vi "TSLIN_LIN_Tab.vi"(7 "Fold Data":bool, 8 "error in (no error)":errorcluster, 9 "Data in":T1 {"REC_Channel" items=["CHN1", "CHN2", "CHN3", "CHN4", "CHN5", "CHN6", "CHN7", "CHN8", "CHN9", "CHN10", "CHN11", "CHN12", "CHN13", "CHN14", "CHN15", "CHN16", "CHN17", "CHN18", "CHN19", "CHN20", "CHN21", "CHN22", "CHN23", "CHN24", "CHN25", "CHN26", "CHN27", "CHN28", "CHN29", "CHN30", "CHN31", "CHN32"]; "LIN_Data"."REC_Channel" items=["CHN1", "CHN2", "CHN3", "CHN4", "CHN5", "CHN6", "CHN7", "CHN8", "CHN9", "CHN10", "CHN11", "CHN12", "CHN13", "CHN14", "CHN15", "CHN16", "CHN17", "CHN18", "CHN19", "CHN20", "CHN21", "CHN22", "CHN23", "CHN24", "CHN25", "CHN26", "CHN27", "CHN28", "CHN29", "CHN30", "CHN31", "CHN32"]; "LIN_Data"."LIN Scheduling Table Array"."LIN_Transmit"."Channel" items=["CHN1", "CHN2", "CHN3", "CHN4", "CHN5", "CHN6", "CHN7", "CHN8", "CHN9", "CHN10", "CHN11", "CHN12", "CHN13", "CHN14", "CHN15", "CHN16", "CHN17", "CHN18", "CHN19", "CHN20", "CHN21", "CHN22", "CHN23", "CHN24", "CHN25", "CHN26", "CHN27", "CHN28", "CHN29", "CHN30", "CHN31", "CHN32"]; "LIN_Data"."LIN Scheduling Table Array"."LIN_Transmit"."ID" format="%.0x"; "LIN_Data"."LIN Scheduling Table Array"."LIN_Transmit"."DLC" format="%.0x"; "LIN_Data"."LIN Scheduling Table Array"."LIN_Transmit"."Set_node_funtiontype" items=["MasterNode", "SlaveNode", "MonitorNote"]; "LIN_Data"."LDF"."LDF loading channel" items=["CHN1", "CHN2", "CHN3", "CHN4", "CHN5", "CHN6", "CHN7", "CHN8", "CHN9", "CHN10", "CHN11", "CHN12", "CHN13", "CHN14", "CHN15", "CHN16", "CHN17", "CHN18", "CHN19", "CHN20", "CHN21", "CHN22", "CHN23", "CHN24", "CHN25", "CHN26", "CHN27", "CHN28", "CHN29", "CHN30", "CHN31", "CHN32"]; "LIN_Data"."LIN_Set_Array"."Set_node_funtiontype" items=["MasterNode", "SlaveNode", "MonitorNote"]; "LIN_Data"."LIN_Set_Array"."Set"."Hardware Type" items=["BUS_UNKNOWN_TYPE", "TS_TCP_DEVICE", "XL_USB_DEVICE", "TS_USB_DEVICE", "PEAK_USB_DEVICE", "KVASER_USB_DEVICE", "ZLG_USB_DEVICE", "ICS_USB_DEVICE", "TS_TC1005_DEVICE", "CANABLE_USB_DEVICE", "TS_WIRELESS_OBD", "TS_USB_DEVICE_EX", "IXXAT_USB_DEVICE", "TS_ETH_IF_DEVICE", "TS_USB_IF_DEVICE", "BUS_DEV_TYPE_COUNT"]; "LIN_Data"."LIN_Set_Array"."Set"."AHwChannel" items=["CHN1", "CHN2", "CHN3", "CHN4", "CHN5", "CHN6", "CHN7", "CHN8", "CHN9", "CHN10", "CHN11", "CHN12", "CHN13", "CHN14", "CHN15", "CHN16", "CHN17", "CHN18", "CHN19", "CHN20", "CHN21", "CHN22", "CHN23", "CHN24", "CHN25", "CHN26", "CHN27", "CHN28", "CHN29", "CHN30", "CHN31", "CHN32"]; "LIN_Data"."LIN_Set_Array"."Set"."AAppChannel" items=["CHN1", "CHN2", "CHN3", "CHN4", "CHN5", "CHN6", "CHN7", "CHN8", "CHN9", "CHN10", "CHN11", "CHN12", "CHN13", "CHN14", "CHN15", "CHN16", "CHN17", "CHN18", "CHN19", "CHN20", "CHN21", "CHN22", "CHN23", "CHN24", "CHN25", "CHN26", "CHN27", "CHN28", "CHN29", "CHN30", "CHN31", "CHN32"]; "LIN_Data"."LIN_Set_Array"."Set"."AProtocol" items=["Lin_Protocol_13", "Lin_Protocol_20", "Lin_Protocol_21", "Lin_Protocol_J2602"]; "LIN_Data"."Funtiontype" items=["MasterNode", "SlaveNode", "MonitorNote"]; "LIN_Data"."LIN_SendHead"."ALINDLC" format="%.0x"; "LIN_Data"."LIN_SendHead"."ALINId" format="%.0x"; "LIN_Data"."LIN_SendHead"."ALINIdxchn" items=["CHN1", "CHN2", "CHN3", "CHN4", "CHN5", "CHN6", "CHN7", "CHN8", "CHN9", "CHN10", "CHN11", "CHN12", "CHN13", "CHN14", "CHN15", "CHN16", "CHN17", "CHN18", "CHN19", "CHN20", "CHN21", "CHN22", "CHN23", "CHN24", "CHN25", "CHN26", "CHN27", "CHN28", "CHN29", "CHN30", "CHN31", "CHN32"]; "LIN_Data"."LIN_Set"."Hardware Type" items=["BUS_UNKNOWN_TYPE", "TS_TCP_DEVICE", "XL_USB_DEVICE", "TS_USB_DEVICE", "PEAK_USB_DEVICE", "KVASER_USB_DEVICE", "ZLG_USB_DEVICE", "ICS_USB_DEVICE", "TS_TC1005_DEVICE", "CANABLE_USB_DEVICE", "TS_WIRELESS_OBD", "TS_USB_DEVICE_EX", "IXXAT_USB_DEVICE", "TS_ETH_IF_DEVICE", "TS_USB_IF_DEVICE", "BUS_DEV_TYPE_COUNT"]; "LIN_Data"."LIN_Set"."AHwChannel" items=["CHN1", "CHN2", "CHN3", "CHN4", "CHN5", "CHN6", "CHN7", "CHN8", "CHN9", "CHN10", "CHN11", "CHN12", "CHN13", "CHN14", "CHN15", "CHN16", "CHN17", "CHN18", "CHN19", "CHN20", "CHN21", "CHN22", "CHN23", "CHN24", "CHN25", "CHN26", "CHN27", "CHN28", "CHN29", "CHN30", "CHN31", "CHN32"]; "LIN_Data"."LIN_Set"."AAppChannel" items=["CHN1", "CHN2", "CHN3", "CHN4", "CHN5", "CHN6", "CHN7", "CHN8", "CHN9", "CHN10", "CHN11", "CHN12", "CHN13", "CHN14", "CHN15", "CHN16", "CHN17", "CHN18", "CHN19", "CHN20", "CHN21", "CHN22", "CHN23", "CHN24", "CHN25", "CHN26", "CHN27", "CHN28", "CHN29", "CHN30", "CHN31", "CHN32"]; "LIN_Data"."LIN_Set"."AProtocol" items=["Lin_Protocol_13", "Lin_Protocol_20", "Lin_Protocol_21", "Lin_Protocol_J2602"]; "LIN_Data"."Channels used" items=["1 Channel"=1, "2 Channels"=2, "3 Channels"=3, "4 Channels"=4, "5 Channels"=5]}, 10 "ALINBuffer":T11[](array[typedef]) {"Properties" format="%x"}, 11 "MulticolumnListbox in":refnum<vi>) -> (3 "Data out":T1 {"REC_Channel" items=["CHN1", "CHN2", "CHN3", "CHN4", "CHN5", "CHN6", "CHN7", "CHN8", "CHN9", "CHN10", "CHN11", "CHN12", "CHN13", "CHN14", "CHN15", "CHN16", "CHN17", "CHN18", "CHN19", "CHN20", "CHN21", "CHN22", "CHN23", "CHN24", "CHN25", "CHN26", "CHN27", "CHN28", "CHN29", "CHN30", "CHN31", "CHN32"]; "LIN_Data"."REC_Channel" items=["CHN1", "CHN2", "CHN3", "CHN4", "CHN5", "CHN6", "CHN7", "CHN8", "CHN9", "CHN10", "CHN11", "CHN12", "CHN13", "CHN14", "CHN15", "CHN16", "CHN17", "CHN18", "CHN19", "CHN20", "CHN21", "CHN22", "CHN23", "CHN24", "CHN25", "CHN26", "CHN27", "CHN28", "CHN29", "CHN30", "CHN31", "CHN32"]; "LIN_Data"."LIN Scheduling Table Array"."LIN_Transmit"."Channel" items=["CHN1", "CHN2", "CHN3", "CHN4", "CHN5", "CHN6", "CHN7", "CHN8", "CHN9", "CHN10", "CHN11", "CHN12", "CHN13", "CHN14", "CHN15", "CHN16", "CHN17", "CHN18", "CHN19", "CHN20", "CHN21", "CHN22", "CHN23", "CHN24", "CHN25", "CHN26", "CHN27", "CHN28", "CHN29", "CHN30", "CHN31", "CHN32"]; "LIN_Data"."LIN Scheduling Table Array"."LIN_Transmit"."ID" format="%.0x"; "LIN_Data"."LIN Scheduling Table Array"."LIN_Transmit"."DLC" format="%.0x"; "LIN_Data"."LIN Scheduling Table Array"."LIN_Transmit"."Set_node_funtiontype" items=["MasterNode", "SlaveNode", "MonitorNote"]; "LIN_Data"."LDF"."LDF loading channel" items=["CHN1", "CHN2", "CHN3", "CHN4", "CHN5", "CHN6", "CHN7", "CHN8", "CHN9", "CHN10", "CHN11", "CHN12", "CHN13", "CHN14", "CHN15", "CHN16", "CHN17", "CHN18", "CHN19", "CHN20", "CHN21", "CHN22", "CHN23", "CHN24", "CHN25", "CHN26", "CHN27", "CHN28", "CHN29", "CHN30", "CHN31", "CHN32"]; "LIN_Data"."LIN_Set_Array"."Set_node_funtiontype" items=["MasterNode", "SlaveNode", "MonitorNote"]; "LIN_Data"."LIN_Set_Array"."Set"."Hardware Type" items=["BUS_UNKNOWN_TYPE", "TS_TCP_DEVICE", "XL_USB_DEVICE", "TS_USB_DEVICE", "PEAK_USB_DEVICE", "KVASER_USB_DEVICE", "ZLG_USB_DEVICE", "ICS_USB_DEVICE", "TS_TC1005_DEVICE", "CANABLE_USB_DEVICE", "TS_WIRELESS_OBD", "TS_USB_DEVICE_EX", "IXXAT_USB_DEVICE", "TS_ETH_IF_DEVICE", "TS_USB_IF_DEVICE", "BUS_DEV_TYPE_COUNT"]; "LIN_Data"."LIN_Set_Array"."Set"."AHwChannel" items=["CHN1", "CHN2", "CHN3", "CHN4", "CHN5", "CHN6", "CHN7", "CHN8", "CHN9", "CHN10", "CHN11", "CHN12", "CHN13", "CHN14", "CHN15", "CHN16", "CHN17", "CHN18", "CHN19", "CHN20", "CHN21", "CHN22", "CHN23", "CHN24", "CHN25", "CHN26", "CHN27", "CHN28", "CHN29", "CHN30", "CHN31", "CHN32"]; "LIN_Data"."LIN_Set_Array"."Set"."AAppChannel" items=["CHN1", "CHN2", "CHN3", "CHN4", "CHN5", "CHN6", "CHN7", "CHN8", "CHN9", "CHN10", "CHN11", "CHN12", "CHN13", "CHN14", "CHN15", "CHN16", "CHN17", "CHN18", "CHN19", "CHN20", "CHN21", "CHN22", "CHN23", "CHN24", "CHN25", "CHN26", "CHN27", "CHN28", "CHN29", "CHN30", "CHN31", "CHN32"]; "LIN_Data"."LIN_Set_Array"."Set"."AProtocol" items=["Lin_Protocol_13", "Lin_Protocol_20", "Lin_Protocol_21", "Lin_Protocol_J2602"]; "LIN_Data"."Funtiontype" items=["MasterNode", "SlaveNode", "MonitorNote"]; "LIN_Data"."LIN_SendHead"."ALINDLC" format="%.0x"; "LIN_Data"."LIN_SendHead"."ALINId" format="%.0x"; "LIN_Data"."LIN_SendHead"."ALINIdxchn" items=["CHN1", "CHN2", "CHN3", "CHN4", "CHN5", "CHN6", "CHN7", "CHN8", "CHN9", "CHN10", "CHN11", "CHN12", "CHN13", "CHN14", "CHN15", "CHN16", "CHN17", "CHN18", "CHN19", "CHN20", "CHN21", "CHN22", "CHN23", "CHN24", "CHN25", "CHN26", "CHN27", "CHN28", "CHN29", "CHN30", "CHN31", "CHN32"]; "LIN_Data"."LIN_Set"."Hardware Type" items=["BUS_UNKNOWN_TYPE", "TS_TCP_DEVICE", "XL_USB_DEVICE", "TS_USB_DEVICE", "PEAK_USB_DEVICE", "KVASER_USB_DEVICE", "ZLG_USB_DEVICE", "ICS_USB_DEVICE", "TS_TC1005_DEVICE", "CANABLE_USB_DEVICE", "TS_WIRELESS_OBD", "TS_USB_DEVICE_EX", "IXXAT_USB_DEVICE", "TS_ETH_IF_DEVICE", "TS_USB_IF_DEVICE", "BUS_DEV_TYPE_COUNT"]; "LIN_Data"."LIN_Set"."AHwChannel" items=["CHN1", "CHN2", "CHN3", "CHN4", "CHN5", "CHN6", "CHN7", "CHN8", "CHN9", "CHN10", "CHN11", "CHN12", "CHN13", "CHN14", "CHN15", "CHN16", "CHN17", "CHN18", "CHN19", "CHN20", "CHN21", "CHN22", "CHN23", "CHN24", "CHN25", "CHN26", "CHN27", "CHN28", "CHN29", "CHN30", "CHN31", "CHN32"]; "LIN_Data"."LIN_Set"."AAppChannel" items=["CHN1", "CHN2", "CHN3", "CHN4", "CHN5", "CHN6", "CHN7", "CHN8", "CHN9", "CHN10", "CHN11", "CHN12", "CHN13", "CHN14", "CHN15", "CHN16", "CHN17", "CHN18", "CHN19", "CHN20", "CHN21", "CHN22", "CHN23", "CHN24", "CHN25", "CHN26", "CHN27", "CHN28", "CHN29", "CHN30", "CHN31", "CHN32"]; "LIN_Data"."LIN_Set"."AProtocol" items=["Lin_Protocol_13", "Lin_Protocol_20", "Lin_Protocol_21", "Lin_Protocol_J2602"]; "LIN_Data"."Channels used" items=["1 Channel"=1, "2 Channels"=2, "3 Channels"=3, "4 Channels"=4, "5 Channels"=5]})   [LabVIEW 2014]
uses:
  Typedef/TLibLIN.ctl
  Typedef/TSLIN_Data.ctl
  Typedef/TSLIN_Config.ctl
  Typedef/TSLIN_SetData.ctl
  All_Control/Typedef/Hardware Type.ctl
  Utilities/Typedef/Hardware_Subtype.ctl
  Typedef/TSLIN_SendHead.ctl
  Typedef/TSLIN_LIN_Set.ctl
  All_Control/Typedef/Blf_Log.ctl
  Typedef/TSLIN_LIN Schedule_Table.ctl
  Typedef/TSLIN_Transmit.ctl
  DataBase/Typedef/CAN/TCANSignal.ctl
  DataBase/Typedef/LIN/TLINSignal.ctl
  DataBase/Typedef/FlexRay/TFlexRaySignal.ctl
  DataBase/Typedef/TDBSignalProperties.ctl
  DataBase/Typedef/TDBFrameProperties.ctl
  DataBase/Typedef/TDBECUProperties.ctl
  DataBase/Typedef/TDBProperties.ctl
  DataBase/Typedef/DataBase_array.ctl
  DataBase/Typedef/DataBase_array_index.ctl
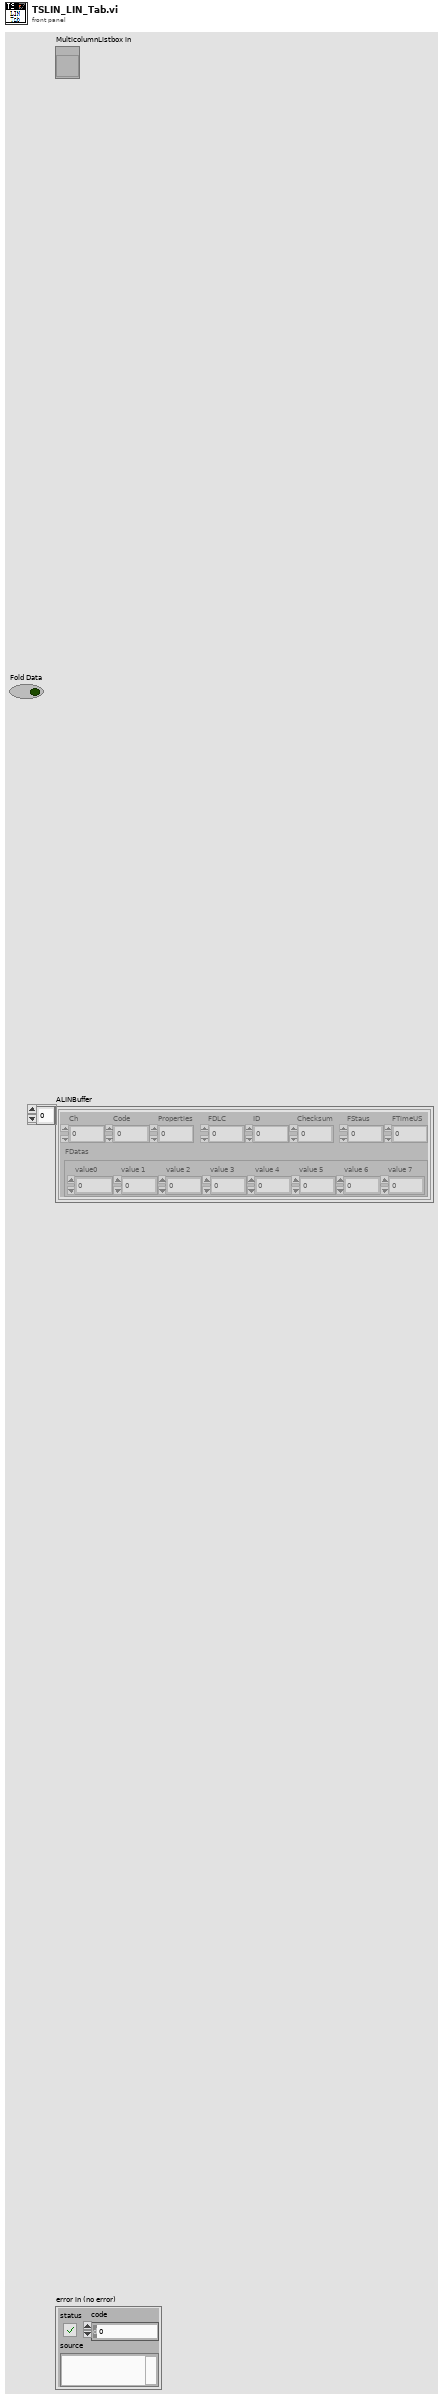
[diagram p1: front panel]
types:
  T1 = typedef "TSLIN_Data.ctl" = cluster{"Communication message":cluster{"Sender":string, "receiver":string, "message":string, "data":variant}, "LIN_Data":T2, "LIN Data array":T11[], "error in":errorcluster, "REC_Channel":i32, "AsynCall?":bool, "DataBase_array":T12}
  T2 = typedef "TSLIN_Config.ctl" = cluster{"DLL_PATH":path, "Channels used":u16, "Funtiontype":i32, "Rx/TX":enum16{"Rx", "Tx"}, "Read message type":enum16{"Only read received messages", "Receive&send messages"}, "async&sync":enum16{"async", "sync"}, "sync_sendTimeout":u16, "LIN_SendHead":T3, "LIN_Set":T4, "LIN_DATA":cluster{"Data0":u8, "Data1":u8, "Data2":u8, "Data3":u8, "Data4":u8, "Data5":u8, "Data6":u8, "Data7":u8}, "LIN_Set_Array":T7[], "LDF":cluster{"LDF Path":path, "LDF loading channel":i32}, "Blf_Log":T8, "LIN Scheduling Table Array":T9[], "REC_Channel":i32}
  T3 = typedef "TSLIN_SendHead.ctl" = cluster{"ALINIdxchn":u8, "ALINId":u32, "ALINDLC":u32}
  T4 = typedef "TSLIN_SetData.ctl" = cluster{"Hardware Type":T5, "Hardware Subtype":T6, "AHwChannel":i32, "AAppChannel":i32, "ABaudrateKbps":sgl, "AProtocol":i32, "AldHW":i32}
  T5 = typedef "Hardware Type.ctl" = i32
  T6 = typedef "Hardware_Subtype.ctl" = enum16{"TS_UNKNOWN_DEVICE", "TSCAN_PRO", "TSCAN_Lite1", "TC1001", "TL1001", "TC1011", "TM5011", "TC1002", "TC1014", "TSCANFD2517", "TC1026", "TC1016", "TC1012", "TC1013", "TLog1002", "TC1034", "TC1018", "GW2116", "TC2115", "MP1013", "TC1113", "TC1114", "TP1013", "TC1017", "TP1018", "TF10XX", "TL1004_FD_4_LIN_2", "TE1051", "TP1051", "TP1034", "TTS9015", "TP1026", "TTS1026", "TTS1034", "TTS1018", "TL1011", "TTS1015_LiAuto", "TTS1013_LiAuto", "TTS1016Pro", "TC1054Pro", "TC1054", "TLog1038", "TO1013", "TC1034Pro", "TC1018Pro", "TC1038Pro", "TS_DEV_END"}
  T7 = typedef "TSLIN_LIN_Set.ctl" = cluster{"Set":T4, "Set_node_funtiontype":i32}
  T8 = typedef "Blf_Log.ctl" = cluster{"Blf_Log_PATH":path}
  T9 = typedef "TSLIN_LIN Schedule_Table.ctl" = cluster{"LIN_Transmit":T10, "Delay(ms)":i32}
  T10 = typedef "TSLIN_Transmit.ctl" = cluster{"Channel":i32, "Rx/TX":enum16{"Rx", "Tx"}, "Set_node_funtiontype":i32, "DLC":u32, "ID":u32, "FDatas":cluster{"value0":u8, "value 1":u8, "value 2":u8, "value 3":u8, "value 4":u8, "value 5":u8, "value 6":u8, "value 7":u8}}
  T11 = typedef "TLibLIN.ctl" = cluster{"Ch":u8, "Code":u8, "Properties":u8, "FDLC":u8, "ID":u8, "Checksum":u8, "FStaus":u8, "FTimeUS":u64, "FDatas":cluster{"value0":u8, "value 1":u8, "value 2":u8, "value 3":u8, "value 4":u8, "value 5":u8, "value 6":u8, "value 7":u8}}
  T12 = typedef "DataBase_array_index.ctl" = refnum<vi>
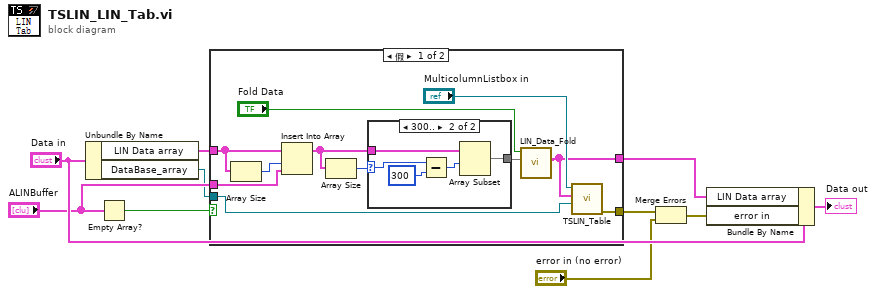
[diagram p0: block diagram]
diagram:
  n1 = Unbundle By Name("Data in") -> ("LIN Data array"=w10:T11[], "DataBase_array"=w1:T12)
  n2 = Empty Array?(array="ALINBuffer") -> (empty?=w7:bool)
  n3 = case shown="假" w7 {
    tunnel: [w12 w28] -> w5
    tunnel: w10 -> [w20 w28]
    tunnel: "ALINBuffer" -> [w19 _]
    tunnel: [w15 _] -> w2
    tunnel: w1 -> [w14 _]
    frame False {
      n4 = Array Size(array=w20) -> (size(s)=w16:i32)
      n5 = Insert Into Array(array=w20, index=w16, new element=w19) -> (w17:T11[])
      n6 = Array Size(array=w17) -> (size(s)=w18:i32)
      n7 = case shown="300.." w18 {
        selector: w18 -> [_ w27]
        tunnel: [w22 w25] -> w13
        tunnel: w17 -> [w22 w23]
        frame 0, Default {
        }
        frame 300.. {
          n8 = Subtract(x=w27, y=300) -> (x-y=w24:i32)
          n9 = Array Subset(array=w23, index=w24) -> (w25:T11[])  [unwired: 1 in]
        }
      }
      n10 = call "LIN_Data_Fold.vi"("LIN Data array"=w13, "Fold Data"="Fold Data") -> ("LIN Data array out"=w12:T11[])  [unwired: 9 in]
      n11 = call "TSLIN_Table.vi"("DataBase_array"=w14, "LIN_Buffer"=w12, "LIN_Data Ref"="MulticolumnListbox in") -> ("错误输出"=w15:errorcluster)  [unwired: 8 in]
    }
    frame True {
    }
  }
  n12 = Merge Errors(w2, "error in (no error)") -> (w3:errorcluster)
  n13 = Bundle By Name(cluster="Data in", "LIN Data array"=w5, "error in"=w3) -> (→"Data out":T1)
